vi "1001_FireAtNoonEveryDay.vi"(8 "error in (no error)":errorcluster) -> (0 "error out":errorcluster)   [LabVIEW 2013]
uses:
  <vilib>/addons/_JKI Toolkits/Caraya/classes/Assert/Assert True.vi
  source/Cron/Create Cron Job.vi
  source/Cron/Compute Next Cron.vi
  source/Cron.Unix/Cron.Unix.lvclass
  <vilib>/addons/_JKI Toolkits/Caraya/classes/Test/Test.lvclass
  <vilib>/addons/_JKI Toolkits/Caraya/classes/Assert/Assert.lvclass
  source/openCron.lvlib
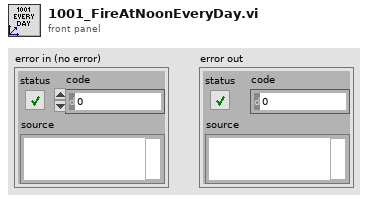
[diagram p1: front panel]
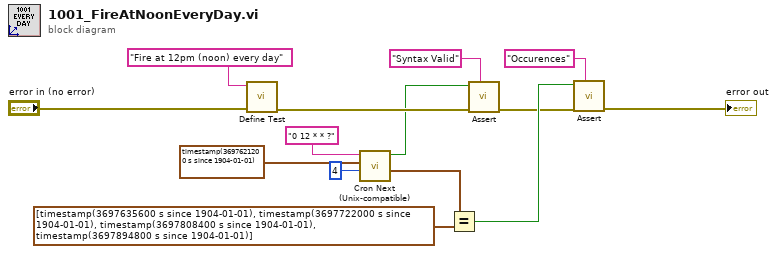
[diagram p0: block diagram]
diagram:
  n1 = call <vilib>:"Define Test.vi"("error in (no error)"="error in (no error)", "Label (VI Title)"="Fire at 12pm (noon) every day") -> ("error out"=w7:errorcluster)  [unwired: 9 in]
  n2 = call "Cron Next (Unix-compatible).vi"("Nb Occurences (min: 1)"=u16 4, "Reference timestamp (Now)"=timestamp(3697621200 s since 1904-01-01) ("y"), "Cron Expression"="0 12 * * ?" ("Expression")) -> ("Occurences"=w2:timestamp[], "syntax valid?"=w1:bool)  [unwired: 6 in, 1 out]
  n3 = Equal?(x=w2, y=timestamp[] [timestamp(3697635600 s since 1904-01-01), timestamp(3697722000 s since 1904-01-01), timestamp(3697808400 s since 1904-01-01), timestamp(3697894800 s since 1904-01-01)]) -> (x = y?=w12:bool)
  n4 = call-poly <vilib>:"Assert.vi"("Label"="Syntax Valid" ("Label (VI Title)"), "error in (no error)"=w7, "True?"=w1) -> ("error out"=w11:errorcluster)  [unwired: 8 in]
  n5 = call-poly <vilib>:"Assert.vi"("Label"="Occurences" ("Label (VI Title)"), "error in (no error)"=w11, "True?"=w12) -> ("error out"=→"error out":errorcluster)  [unwired: 8 in]
